vi "CLD 12 CSV file commands utility.vi"(8 "Fehler (Eingang)":T3) -> (0 "Fehler (Ausgang)":T3, 3 "Befehls-Ausgangs-Array":T1[](array[typedef]))   [LabVIEW 2014]
doc: "CLD 12 - Utility für Dateizugriff. Dieses VI wandelt den Textbefehl in das entsprechende Enum-Element um."
uses:
  CLD 12 Data Cluster.ctl
  CLD 12 Sequencer Enum.ctl
  <vilib>/Utility/file.llb/Read From Spreadsheet File (string).vi
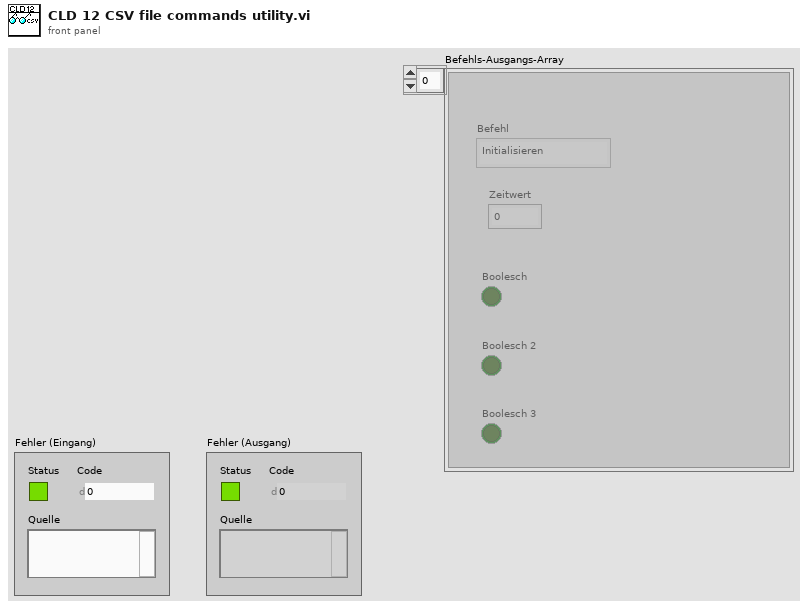
[diagram p1: front panel]
types:
  T1 = typedef "CLD 12 Data Cluster.ctl" = cluster{"Befehl":T2, "Zeitwert":dbl, "Boolesch":bool, "Boolesch 2":bool, "Boolesch 3":bool}
  T2 = typedef "CLD 12 Sequencer Enum.ctl" = enum16{"Initialisieren", "SetTime", "RunState1", "Runstate2", "Ruhezustand", "Starten"}
  T3 = cluster{"Status":bool, "Code":i32, "Quelle":string}
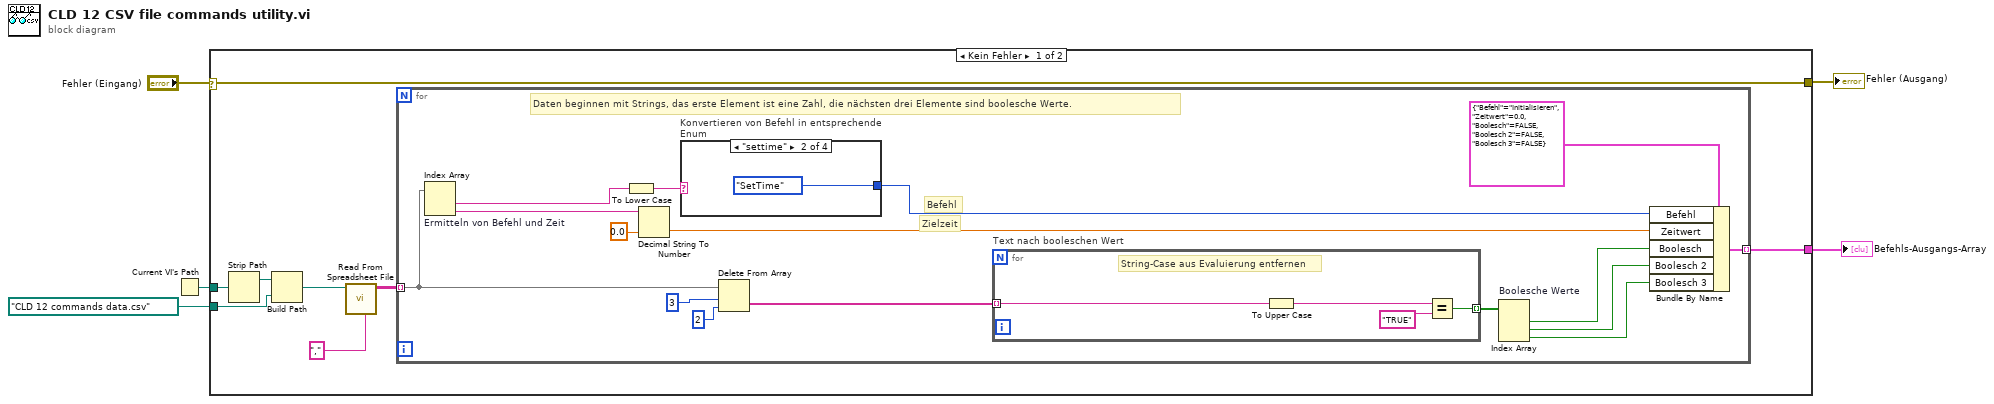
[diagram p0: block diagram]
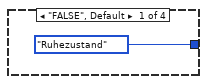
[diagram p2: hidden frame]
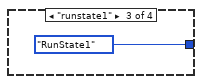
[diagram p3: hidden frame]
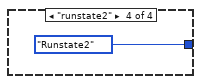
[diagram p4: hidden frame]
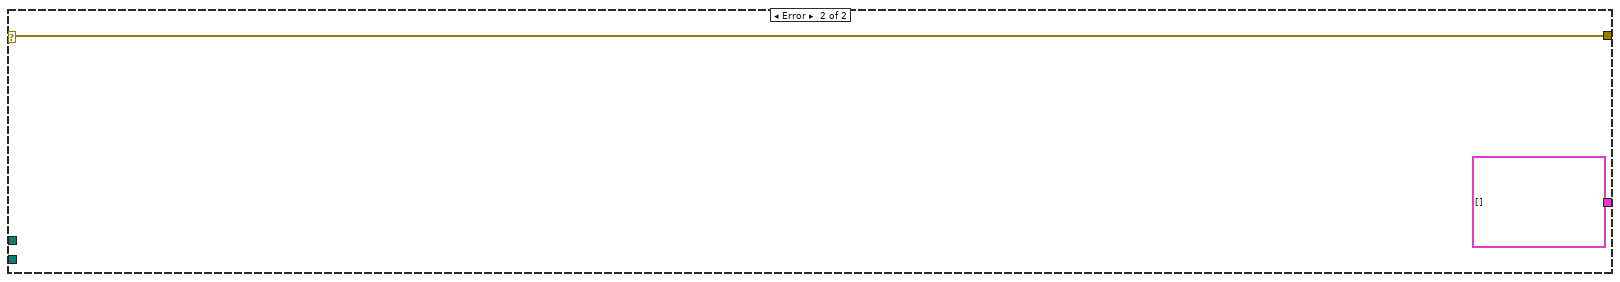
[diagram p5: hidden frame]
diagram:
  n1 = Current VI's Path() -> (path=w2:path)
  n2 = case shown="Kein Fehler" "Fehler (Eingang)" {
    selector: "Fehler (Eingang)" -> [w13 w39]
    tunnel: [w10 T1[] []] -> w1
    tunnel: path "CLD 12 commands data.csv" -> [w8 _]
    tunnel: w2 -> [w9 _]
    tunnel: [w13 w39] -> w3
    frame No Error {
      n3 = Strip Path(path=w9) -> (stripped path=w6:path)  [unwired: 1 out]
      n4 = Build Path(base path=w6, name or relative path=w8) -> (appended path=w7:path)
      n5 = call-poly <vilib>:"Read From Spreadsheet File.vi"("delimiter (\\t)"="," ("Trennzeichen (\\t)"), "file path (dialog if empty)"=w7) -> ("all rows"=w12:string[][])  [unwired: 5 in, 4 out]
      n6 = for {
        tunnel: w12 -> [w29] mode=indexing
        tunnel: [w21] -> w10 mode=indexing
        # "Zielzeit"
        # "Befehl"
        # "Daten beginnen mit Strings, das erste Element ist eine Zahl, die nächsten drei Elemente sind boolesche Werte."
        n7 = Index Array "Ermitteln von Befehl und Zeit"(array=w29) -> (element #1=w17:string, element #2=w20:string)  [unwired: 2 in]
        n8 = To Lower Case(string=w17) -> (all lower case string=w15:string)
        n9 = Decimal String To Number(string=w20, default (0L)=0.0) -> (number=w19:dbl)  [unwired: 1 in, 1 out]
        n10 = case "Konvertieren von Befehl in entsprechende Enum" shown="\"settime\"" w15 {
          tunnel: [CLD_12_Sequencer_Enum."Ruhezustand" ("Befehl") CLD_12_Sequencer_Enum."SetTime" ("Befehl") CLD_12_Sequencer_Enum."RunState1" ("Befehl") CLD_12_Sequencer_Enum."Runstate2" ("Befehl")] -> w16
          frame "FALSE", Default {
          }
          frame "settime" {
          }
          frame "runstate1" {
          }
          frame "runstate2" {
          }
        }
        n11 = Delete From Array(array=w29, length=3 ("Länge"), index=2 ("Index")) -> (deleted portion=w14:string[])  [unwired: 1 out]
        n12 = for "Text nach booleschen Wert" {
          tunnel: w14 -> [w37] mode=indexing
          tunnel: [w34] -> w26 mode=indexing
          # "String-Case aus Evaluierung entfernen"
          n13 = To Upper Case(1:w37) -> (0:w36:string)
          n14 = Equal?(x=w36, y="TRUE") -> (x = y?=w34:bool)
        }
        n15 = Index Array "Boolesche Werte"(array=w26) -> (element #1=w24:bool, element #2=w23:bool, element #3=w22:bool)  [unwired: 3 in]
        n16 = Bundle By Name(cluster=T1 {"Befehl"=enum."Initialisieren", "Zeitwert"=0.0, "Boolesch"=FALSE, "Boolesch 2"=FALSE, "Boolesch 3"=FALSE} ("CLD 12 - Daten-Cluster"), "Befehl"=w16, "Zeitwert"=w19, "Boolesch"=w24, "Boolesch 2"=w23, "Boolesch 3"=w22) -> (w21:T1)
      }
    }
    frame Error {
    }
  }
  "Fehler (Ausgang)" <- w3
  "Befehls-Ausgangs-Array" <- w1
